vi "RFFE Main Control.vi"(7 "RFFE Function":enum16{"Write", "Read"}(ring), 8 "Error In":errorcluster, 9 "Reg_Address_Data":T1={"Address"=81, "Data"=0} {"Address" format="%.0x"}, 10 "USID":T2 max=15, 11 "HSDIO Sessions":T3) -> (0 "Error Out":errorcluster, 1 "Converted Data":cluster{"USID":u8, "Register":u8, "Data":u8} {"Register" max=31 format="%.0x"; "USID" max=15 format="%.0x"}, 2 "Data_Readback":u8[](array[numeric])=[31, 144, 7], 3 "Registers_Readback":i32[](array[numeric]), 5 "HSDIO":digitalwaveform(graph)={"t0"=timestamp(3585852840.1106524 s since 1904-01-01), "dt"=5e-07, "Y"={"transitions"=[], "data"=[[1, 0, 1, 0], [1, 0, 1, 0], [1, 0, 1, 0], [1, 0, 1, 0], [1, 0, 1, 0], [1, 0, 1, 0], [1, 0, 1, 0], [1, 0, 1, 0], [0, 0, 0, 0], [0, 0, 0, 0], [0, 0, 0, 0], [0, 0, 0, 0], [0, 0, 0, 0], [0, 0, 0, 0], [0, 0, 0, 0], [0, 0, 0, 0], [0, 1, 0, 1], [0, 1, 0, 1], [0, 1, 0, 1], [0, 1, 0, 1], [0, 0, 0, 0], [0, 0, 0, 0], [0, 0, 0, 0], [0, 0, 0, 0], [1, 1, 1, 1], [1, 1, 1, 1], [1, 1, 1, 1], [1, 1, 1, 1], [1, 0, 1, 0], [1, 0, 1, 0], [1, 0, 1, 0], [1, 0, 1, 0], [1, 1, 1, 1], [1, 1, 1, 1], [1, 1, 1, 1], [1, 1, 1, 1], [1, 0, 1, 0], [1, 0, 1, 0], [1, 0, 1, 0], [1, 0, 1, 0], [0, 1, 0, 1], [0, 1, 0, 1], [0, 1, 0, 1], [0, 1, 0, 1], [0, 0, 0, 0], [0, 0, 0, 0], [0, 0, 0, 0], [0, 0, 0, 0], [0, 1, 0, 1], [0, 1, 0, 1], [0, 1, 0, 1], [0, 1, 0, 1], [0, 0, 0, 0], [0, 0, 0, 0], [0, 0, 0, 0], [0, 0, 0, 0], [1, 1, 1, 1], [1, 1, 1, 1], [1, 1, 1, 1], [1, 1, 1, 1], [1, 0, 1, 0], [1, 0, 1, 0], [1, 0, 1, 0], [1, 0, 1, 0], [0, 1, 0, 1], [0, 1, 0, 1], [0, 1, 0, 1], [0, 1, 0, 1], [0, 0, 0, 0], [0, 0, 0, 0], [0, 0, 0, 0], [0, 0, 0, 0], [1, 1, 1, 1], [1, 1, 1, 1], [1, 1, 1, 1], [1, 1, 1, 1], [1, 0, 1, 0], [1, 0, 1, 0], [1, 0, 1, 0], [1, 0, 1, 0], [1, 1, 1, 1], [1, 1, 1, 1], [1, 1, 1, 1], [1, 1, 1, 1], [1, 0, 1, 0], [1, 0, 1, 0], [1, 0, 1, 0], [1, 0, 1, 0], [1, 1, 1, 1], [1, 1, 1, 1], [1, 1, 1, 1], [1, 1, 1, 1], [1, 0, 1, 0], [1, 0, 1, 0], [1, 0, 1, 0], [1, 0, 1, 0], [0, 1, 0, 1], [0, 1, 0, 1], [0, 1, 0, 1], [0, 1, 0, 1], [0, 0, 0, 0], [0, 0, 0, 0], [0, 0, 0, 0], [0, 0, 0, 0], [0, 1, 0, 1], [0, 1, 0, 1], [0, 1, 0, 1], [0, 1, 0, 1], [0, 0, 0, 0], [0, 0, 0, 0], [0, 0, 0, 0], [0, 0, 0, 0], [1, 1, 1, 1], [1, 1, 1, 1], [1, 1, 1, 1], [1, 1, 1, 1], [1, 0, 1, 0], [1, 0, 1, 0], [1, 0, 1, 0], [1, 0, 1, 0], [1, 1, 1, 1], [1, 1, 1, 1], [1, 1, 1, 1], [1, 1, 1, 1], [1, 0, 1, 0], [1, 0, 1, 0], [1, 0, 1, 0], [1, 0, 1, 0], [0, 1, 0, 1], [0, 1, 0, 1], [0, 1, 0, 1], [0, 1, 0, 1], [0, 0, 0, 0], [0, 0, 0, 0], [0, 0, 0, 0], [0, 0, 0, 0], [0, 1, 0, 1], [0, 1, 0, 1], [0, 1, 0, 1], [0, 1, 0, 1], [0, 0, 0, 0], [0, 0, 0, 0], [0, 0, 0, 0], [0, 0, 0, 0], [0, 1, 0, 1], [0, 1, 0, 1], [0, 1, 0, 1], [0, 1, 0, 1], [0, 0, 0, 0], [0, 0, 0, 0], [0, 0, 0, 0], [0, 0, 0, 0], [0, 1, 0, 1], [0, 1, 0, 1], [0, 1, 0, 1], [0, 1, 0, 1], [0, 0, 0, 0], [0, 0, 0, 0], [0, 0, 0, 0], [0, 0, 0, 0], [0, 1, 0, 1], [0, 1, 0, 1], [0, 1, 0, 1], [0, 1, 0, 1], [0, 0, 0, 0], [0, 0, 0, 0], [0, 0, 0, 0], [0, 0, 0, 0], [0, 1, 0, 1], [0, 1, 0, 1], [0, 1, 0, 1], [0, 1, 0, 1], [0, 0, 0, 0], [0, 0, 0, 0], [0, 0, 0, 0], [0, 0, 0, 0], [0, 1, 0, 1], [0, 1, 0, 1], [0, 1, 0, 1], [0, 1, 0, 1], [0, 0, 0, 0], [0, 0, 0, 0], [0, 0, 0, 0], [0, 0, 0, 0], [0, 1, 0, 1], [0, 1, 0, 1], [0, 1, 0, 1], [0, 1, 0, 1], [0, 0, 0, 0], [0, 0, 0, 0], [0, 0, 0, 0], [0, 0, 0, 0], [0, 1, 0, 1], [0, 1, 0, 1], [0, 1, 0, 1], [0, 1, 0, 1], [0, 0, 0, 0], [0, 0, 0, 0], [0, 0, 0, 0], [0, 0, 0, 0], [1, 0, 1, 0], [1, 0, 1, 0], [1, 0, 1, 0], [1, 0, 1, 0], [1, 0, 1, 0], [1, 0, 1, 0], [1, 0, 1, 0], [1, 0, 1, 0], [0, 0, 0, 0], [0, 0, 0, 0], [0, 0, 0, 0], [0, 0, 0, 0], [0, 0, 0, 0], [0, 0, 0, 0], [0, 0, 0, 0], [0, 0, 0, 0], [0, 1, 0, 1], [0, 1, 0, 1], [0, 1, 0, 1], [0, 1, 0, 1], [0, 0, 0, 0], [0, 0, 0, 0], [0, 0, 0, 0], [0, 0, 0, 0], [1, 1, 1, 1], [1, 1, 1, 1], [1, 1, 1, 1], [1, 1, 1, 1], [1, 0, 1, 0], [1, 0, 1, 0], [1, 0, 1, 0], [1, 0, 1, 0], [1, 1, 1, 1], [1, 1, 1, 1], [1, 1, 1, 1], [1, 1, 1, 1], [1, 0, 1, 0], [1, 0, 1, 0], [1, 0, 1, 0], [1, 0, 1, 0], [0, 1, 0, 1], [0, 1, 0, 1], [0, 1, 0, 1], [0, 1, 0, 1], [0, 0, 0, 0], [0, 0, 0, 0], [0, 0, 0, 0], [0, 0, 0, 0], [0, 1, 0, 1], [0, 1, 0, 1], [0, 1, 0, 1], [0, 1, 0, 1], [0, 0, 0, 0], [0, 0, 0, 0], [0, 0, 0, 0], [0, 0, 0, 0], [1, 1, 1, 1], [1, 1, 1, 1], [1, 1, 1, 1], [1, 1, 1, 1], [1, 0, 1, 0], [1, 0, 1, 0], [1, 0, 1, 0], [1, 0, 1, 0], [1, 1, 1, 1], [1, 1, 1, 1], [1, 1, 1, 1], [1, 1, 1, 1], [1, 0, 1, 0], [1, 0, 1, 0], [1, 0, 1, 0], [1, 0, 1, 0], [1, 1, 1, 1], [1, 1, 1, 1], [1, 1, 1, 1], [1, 1, 1, 1], [1, 0, 1, 0], [1, 0, 1, 0], [1, 0, 1, 0], [1, 0, 1, 0], [1, 1, 1, 1], [1, 1, 1, 1], [1, 1, 1, 1], [1, 1, 1, 1], [1, 0, 1, 0], [1, 0, 1, 0], [1, 0, 1, 0], [1, 0, 1, 0], [1, 1, 1, 1], [1, 1, 1, 1], [1, 1, 1, 1], [1, 1, 1, 1], [1, 0, 1, 0], [1, 0, 1, 0], [1, 0, 1, 0], [1, 0, 1, 0], [0, 1, 0, 1], [0, 1, 0, 1], [0, 1, 0, 1], [0, 1, 0, 1], [0, 0, 0, 0], [0, 0, 0, 0], [0, 0, 0, 0], [0, 0, 0, 0], [0, 1, 0, 1], [0, 1, 0, 1], [0, 1, 0, 1], [0, 1, 0, 1], [0, 0, 0, 0], [0, 0, 0, 0], [0, 0, 0, 0], [0, 0, 0, 0], [0, 1, 0, 1], [0, 1, 0, 1], [0, 1, 0, 1], [0, 1, 0, 1], [0, 0, 0, 0], [0, 0, 0, 0], [0, 0, 0, 0], [0, 0, 0, 0], [0, 1, 0, 1], [0, 1, 0, 1], [0, 1, 0, 1], [0, 1, 0, 1], [0, 0, 0, 0], [0, 0, 0, 0], [0, 0, 0, 0], [0, 0, 0, 0], [1, 1, 5, 1], [1, 1, 5, 1], [1, 1, 5, 1], [1, 1, 5, 1], [1, 0, 4, 0], [1, 0, 5, 0], [1, 0, 5, 0], [1, 0, 5, 0], [0, 1, 5, 1], [0, 1, 5, 1], [0, 1, 5, 1], [0, 1, 5, 1], [0, 0, 3, 0], [0, 0, 5, 0], [0, 0, 5, 0], [0, 0, 5, 0], [0, 1, 5, 1], [0, 1, 5, 1], [0, 1, 5, 1], [0, 1, 5, 1], [0, 0, 3, 0], [0, 0, 5, 0], [0, 0, 5, 0], [0, 0, 5, 0], [0, 1, 5, 1], [0, 1, 5, 1], [0, 1, 5, 1], [0, 1, 5, 1], [0, 0, 3, 0], [0, 0, 5, 0], [0, 0, 5, 0], [0, 0, 5, 0], [0, 1, 5, 1], [0, 1, 5, 1], [0, 1, 5, 1], [0, 1, 5, 1], [0, 0, 3, 0], [0, 0, 5, 0], [0, 0, 5, 0], [0, 0, 5, 0], [0, 1, 5, 1], [0, 1, 5, 1], [0, 1, 5, 1], [0, 1, 5, 1], [0, 0, 3, 0], [0, 0, 5, 0], [0, 0, 5, 0], [0, 0, 5, 0], [0, 1, 5, 1], [0, 1, 5, 1], [0, 1, 5, 1], [0, 1, 5, 1], [0, 0, 3, 0], [0, 0, 5, 0], [0, 0, 5, 0], [0, 0, 5, 0], [0, 1, 5, 1], [0, 1, 5, 1], [0, 1, 5, 1], [0, 1, 5, 1], [0, 0, 3, 0], [0, 0, 5, 0], [0, 0, 5, 0], [0, 0, 5, 0], [0, 1, 5, 1], [0, 1, 5, 1], [0, 1, 5, 1], [0, 1, 5, 1], [0, 0, 3, 0], [0, 0, 5, 0], [0, 0, 5, 0], [0, 0, 5, 0], [0, 1, 0, 1], [0, 1, 0, 1], [0, 1, 0, 1], [0, 1, 0, 1], [0, 0, 0, 0], [0, 0, 0, 0], [0, 0, 0, 0], [0, 0, 0, 0]]}})   [LabVIEW 2013]
uses:
  Controls/USID.ctl
  Controls/Reg_Address_Data.ctl
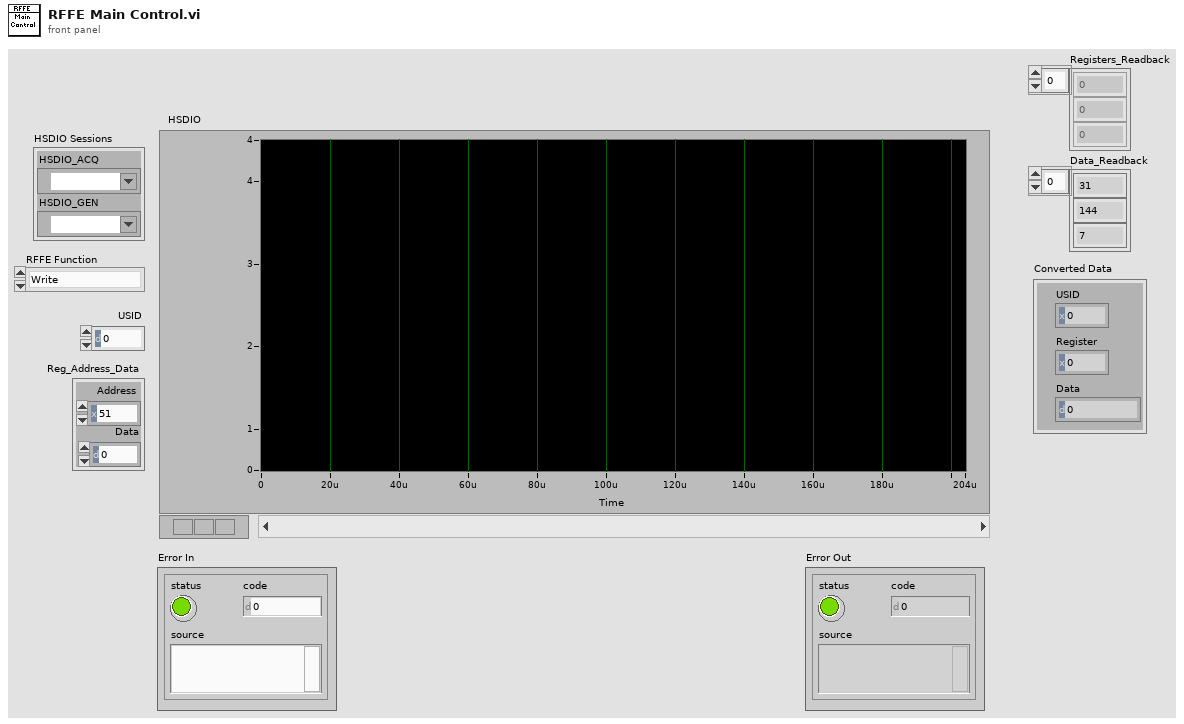
[diagram p1: front panel]
types:
  T1 = typedef "Reg_Address_Data.ctl" = cluster{"Address":u8, "Data":u8}
  T2 = typedef "USID.ctl" = u8
  T3 = cluster{"HSDIO_ACQ":refnum<k15>, "HSDIO_GEN":refnum<k15>}
  T4 = cluster{"Slave Address":u8, "Register":u8, "Data":u8}
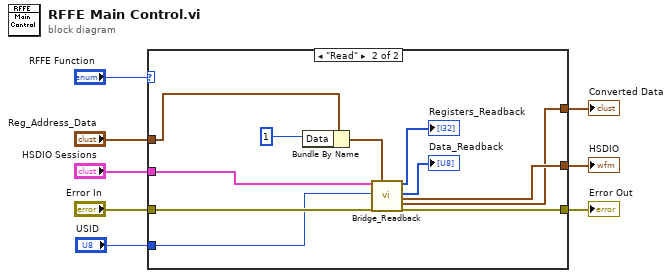
[diagram p0: block diagram]
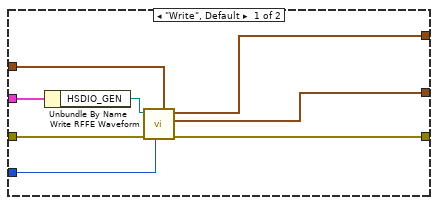
[diagram p2: hidden frame]
diagram:
  n1 = case shown="\"Read\"" "RFFE Function" {
    tunnel: "HSDIO Sessions" -> [w16 w27]
    tunnel: [w14 w24] -> w6
    tunnel: "Error In" -> [w13 w26]
    tunnel: [w12 w25] -> w4
    tunnel: "USID" -> [w11 w23]
    tunnel: "Reg_Address_Data" -> [w10 w19]
    tunnel: [w9 w22] -> w1
    frame "Write", Default {
      n2 = Unbundle By Name(w16) -> ("HSDIO_GEN"=w15:refnum<k15>)
      n3 = call "Write RFFE Waveform.vi"("Reg_Address_Data"=w10, "USID"=w11, "error in (no error)"=w13, "instrument handle"=w15) -> ("error out"=w12:errorcluster, "Digital Waveform Graph"=w14:digitalwaveform, "Converted Data"=w9:cluster{"USID":u8, "Register":u8, "Data":u8})  [unwired: 5 in]
    }
    frame "Read" {
      n4 = Bundle By Name(cluster=w19, "Data"=u8 1) -> (w18:T1)
      n5 = call "Bridge_Readback.vi"("HSDIO Sessions"=w27, "USID"=w23, "Error In"=w26, "Reg_Address_to_Read"=w18) -> ("Registers_Readback"=→"Registers_Readback":i32[], "Data_Readback"=→"Data_Readback":u8[], "Waveform Graph"=w24:digitalwaveform, "Converted Data"=w22:T4, "Error Out"=w25:errorcluster)  [unwired: 11 in]
    }
  }
  "HSDIO" <- w6
  "Error Out" <- w4
  "Converted Data" <- w1
